vi "Update from Double.vi"(6 "Timestamp (Now)":dbl, 7 "precision (6)":i16, 8 "error in (no error)":errorcluster, 10 "Double":dbl, 11 "StringChannel in":refnum<class "StringChannel.lvclass">) -> (0 "error out":errorcluster, 3 "StringChannel out":refnum<class "StringChannel.lvclass">)   [LabVIEW 2020, in "Vecto.lvlib" / "StringChannel.lvclass"]
uses:
  StringChannel.lvclass
  StringChannel.lvclass/StringChannel.ctl
  StringGroup/StringGroup.lvclass
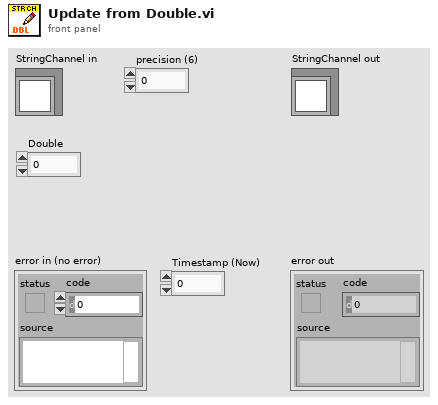
[diagram p1: front panel]
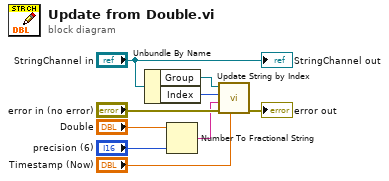
[diagram p0: block diagram]
diagram:
  n1 = Unbundle By Name("StringChannel in") -> ("Group"=w5:refnum<class "StringGroup.lvclass">, "Index"=w6:i32)
  n2 = Number To Fractional String(number="Double", precision (6)="precision (6)") -> (F-format string=w1:string)  [unwired: 2 in]
  n3 = call "Update String by Index.vi"("Timestamp (Now)"="Timestamp (Now)", "error in (no error)"="error in (no error)", "String"=w1, "Index"=w6, "StringGroup in"=w5) -> ("error out"=→"error out":errorcluster)  [unwired: 5 in, 1 out]
  "StringChannel out" <- "StringChannel in"
